vi "Get New Filepath.vi"(2 "Selected Template VI or CTL name (including file extension)":string, 3 "New Filename":string, 4 "Destination Folder":path) -> (0 "Validated Filename of VI or CTL to be created (including extension)":string, 1 "Filepath of VI or CTL to be created":path)   [LabVIEW 2022 SP3]
doc: "This VI creates the filename, and filepath for the VI or CTL to be created."
panel:
  # "Development\nControls or indicators that are useful for development or testing, but which are not outputs of the VI."
  # "Input\nInputs to the VI"
  # "Output\nOutputs of the VI"
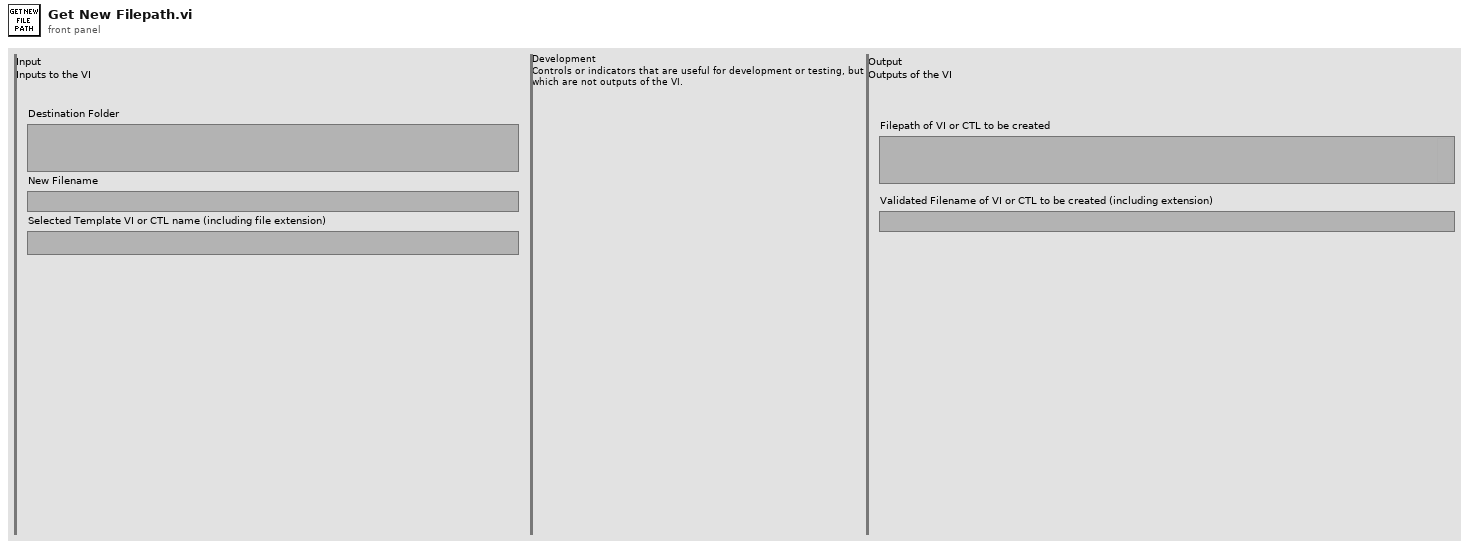
[diagram p1: front panel]
types:
  T1 = typedef "Output File Extension (enum).ctl" = enum16{".vi", ".ctl"}
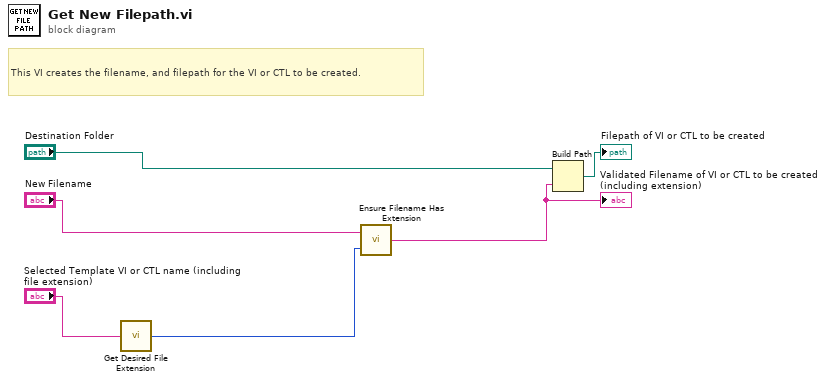
[diagram p0: block diagram]
diagram:
  # "This VI creates the filename, and filepath for the VI or CTL to be created."
  n1 = call "Get Desired File Extension.vi"("Selected Template VI or CTL name (including file extension)"="Selected Template VI or CTL name (including file extension)") -> ("Desired File Extension"=w4:T1)
  n2 = call "Ensure Filename Has Extension.vi"("Desired File Extension"=w4, "Filename (with or without extension)"="New Filename") -> ("Filename With Extension"=w1:string)
  "Validated Filename of VI or CTL to be created (including extension)" <- w1
  n3 = Build Path(base path="Destination Folder", name or relative path=w1) -> (appended path=→"Filepath of VI or CTL to be created":path)
